vi "motor init.vi"(6 "PID":cluster{"Kp":dbl, "Ki":dbl, "Kd":dbl}, 7 "Variable PID(Kp)":T1, 8 "Error In":errorcluster, 9 "dt(s)":dbl, 10 "Enum":T3, 11 "Motor single.lvclass":refnum<class "Motor single.lvclass">) -> (0 "Error Out":errorcluster, 3 "output object":refnum<class "Motor single.lvclass">)   [LabVIEW 2019, in "Motor single.lvclass"]
uses:
  Motor single.lvclass
  motor enum(FPGA).ctl
  Variable PID(Kp).ctl
  Variable PID(Kp) mode enum.ctl
  motor control & config.ctl
  Motor single.lvclass/Motor single.ctl
  FPGA/FPGA varible.vi
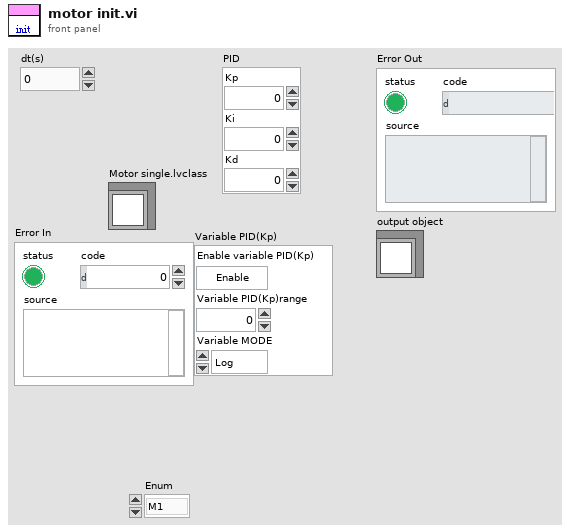
[diagram p1: front panel]
types:
  T1 = typedef "Motor single.lvclass/Variable PID(Kp).ctl" = cluster{"Enable variable PID(Kp)":bool, "Variable PID(Kp)range":dbl, "Variable MODE":T2}
  T2 = typedef "Motor single.lvclass/Variable PID(Kp) mode enum.ctl" = enum16{"Log", "Sin&Cos", "Linear", "reverse Log", "const"}
  T3 = typedef "Motor single.lvclass/motor enum(FPGA).ctl" = enum16{"M1", "M2", "M3", "M4"}
  T4 = typedef "Motor single.lvclass/motor control & config.ctl" = enum16{"control", "config"}
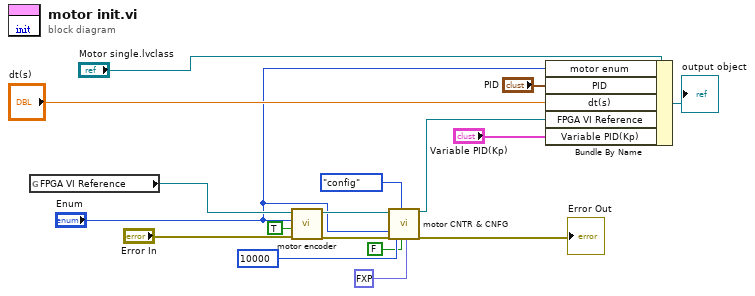
[diagram p0: block diagram]
diagram:
  n1 = global read "FPGA varible.vi" "FPGA VI Reference"() -> (w14:refnum<k20>)
  n2 = call "motor encoder.vi"("Error In"="Error In", "Motor Reset"=TRUE, "Motor Enum"="Enum", "FPGA VI Reference In"=w14) -> ("Error Out"=w9:errorcluster, "FPGA VI Reference Out"=w7:refnum<k20>)  [unwired: 5 in, 1 out]
  n3 = call "motor CNTR & CNFG.vi"("FPGA VI Reference"=w7, "Motor select"="Enum", "Error In"=w9, "Motor period"=i64 10000, "Function"=motor_control_&_config."config", "Motor.enable_divider"=FALSE, "Motor.divider"=fxp<+,4,4> 0.0) -> ("FPGA VI Reference Out"=w6:refnum<k20>, "error out"=→"Error Out":errorcluster)  [unwired: 10 in, 1 out]
  n4 = Bundle By Name(cluster="Motor single.lvclass", "motor enum"="Enum", "PID"="PID", "dt(s)"="dt(s)", "FPGA VI Reference"=w6, "Variable PID(Kp)"="Variable PID(Kp)") -> (→"output object":refnum<class "Motor single.lvclass">)
